vi "Read Binary Data.vi"(8 "error in (no error)":errorcluster, 9 "timeout ms (5000)":i32=5000, 11 "WebSocket in":refnum<class "WebSocket.lvclass">) -> (0 "error out":errorcluster, 2 "Data":u8[](array[numeric]), 3 "WebSocket out":refnum<class "WebSocket.lvclass">)   [LabVIEW 2021, in "WebSockets.lvlib" / "WebSocket.lvclass"]
doc: "Reads a binary frame from a WebSocket connection endpoint. Internally handles fragmented messages and Ping requests.\n\nIf a text frame is received, the data will be returned and a warning generated.\nWebSockets 2.0.1.40\nSam Sharp - MediaMongrels Ltd\nCopyright (c) 2019, MediaMongrels Ltd"
uses:
  WebSocket.lvclass
  WebSocket.lvclass/WebSocket.ctl
  Timing/Calculate Timeout.vi
  Low-Level Read.vi
  Pong.vi
  Timing/Tick Count with Error Wires.vi
  Socket Read.vi
  Low-Level Write.vi
  DataLengthBytes.vi
  EncodeMaskedBytes.vi
  Socket Write.vi
  DecodeMaskedBytes.vi
  Sockets/Socket/Socket.lvclass
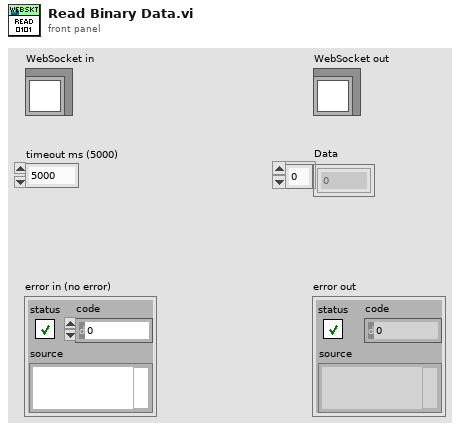
[diagram p1: front panel]
types:
  T1 = typedef "WebSockets.lvlib/WebSocket.lvclass/Opcodes.ctl" = u8
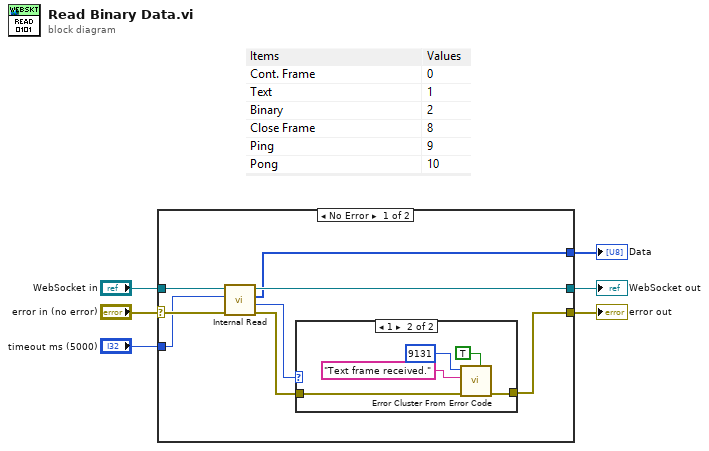
[diagram p0: block diagram]
diagram:
  n1 = case shown="No Error" "error in (no error)" {
    selector: "error in (no error)" -> [w13 w22]
    tunnel: [w9 w22] -> w5
    tunnel: [w10 w21] -> w3
    tunnel: "WebSocket in" -> [w14 w21]
    tunnel: "timeout ms (5000)" -> [w12 _]
    tunnel: [w7 _] -> w1
    frame No Error {
      n2 = call "Internal Read.vi"("error in (no error)"=w13, "timeout ms"=w12, "WebSocket in"=w14) -> ("error out"=w11:errorcluster, "Opcode"=w8:T1, "Data"=w7:u8[], "WebSocket out"=w10:refnum<class "WebSocket.lvclass">)  [unwired: 5 in]
      n3 = case shown="1" w8 {
        tunnel: w11 -> [w15 w20]
        tunnel: [w15 w16] -> w9
        frame Default {
        }
        frame 1 {
          n4 = call <vilib>:"Error Cluster From Error Code.vi"("is warning? (False)"=TRUE, "error in (no error)"=w20, "error message (\"\")"="Text frame received." ("error message (\"\")"), "error code (0)"=9131) -> ("error out"=w16:errorcluster)  [unwired: 5 in]
        }
      }
    }
    frame Error {
    }
  }
  "error out" <- w5
  "WebSocket out" <- w3
  "Data" <- w1
